vi "LabviewMonitoringApplicationFullDataFromCloud.vi"() -> ()   [LabVIEW 2024]
uses:
  <vilib>/Utility/error.llb/Trim Whitespace One-Sided.vi
  <vilib>/Instr/_visa.llb/VISA Configure Serial Port (Instr).vi
  <vilib>/Utility/file.llb/Read Delimited Spreadsheet (DBL).vi
  <vilib>/regexp/Match Regular Expression.xnode
  <vilib>/httpClient/LabVIEWHTTPClient.lvlib
  <vilib>/JDP Science/JSONtext/JSONtext.lvlib
panel:
  out "body":string
  out "CONTROL PANEL":enum32{"DASHBOARD", "Settings"}(tab)
  out "HISTORICAL DATA":dbl[][](graph)
  in  "To":string
  in  "From":string
  in  "Date":string
  in  "OK Button":bool
  in  "C/F":bool
  out "Pericol pentru sanatate":u32(colorbox)
  out "Disconfort sever":u32(colorbox)
  out "Disconfort moderat":u32(colorbox)
  out "Usor discomfort":u32(colorbox)
  out "Confortabil":u32(colorbox)
  out "Snapshot data":string
  out "Waveform Chart":T1(graph) caption="LIVE DATA"
  out "return count read":u32
  in  "STOP":bool=TRUE
  in  "milliseconds to wait":u32=1000
  out "VISA resource name out read":refnum<visa-resource-name>="COM32"
  in  "Start Measurement":bool=TRUE
  out "READ BUFFER":string
  out "Prog. Cnt":i64
  out "AdcValue":dbl
  out "R0 value (kOHm)":dbl(slide) scale=0.0..10.0 scale format="%.2f"
  out "Volatge":dbl(knob) scale=0.0..3.3
  out "Temperature °C":dbl(slide) scale=0.0..100.0 scale format="%#.2g"
  out "Humidity %":dbl(knob) scale=0.1..100.0 scale format="%#.2g"
  out "Heat Index":dbl(slide) scale=0.0..100.0
  out "iPPM_Smoke":i64(slide) scale=0.0..500.0
  out "iPPM_LPG":i64(slide) scale=0.0..100.0
  out "iPPM_CO":i64(slide) scale=0.0..400.0
  in  "Live Data / Historical Data":bool=TRUE
  in  "Temperature":bool=TRUE
  in  "Humidity":bool=TRUE
  in  "PMM_CO":bool=TRUE
  in  "HeatIndex":bool=TRUE
  in  "PMM_LPG":bool=TRUE
  in  "PMM_Smoke":bool=TRUE
  in  "Save file":bool
  in  "file path (use dialog)":path
  out "ITU":dbl format="%#.2g"
  in  "file path (dialog if empty)":path
  out "error out read  from VISA":errorcluster={"status"=TRUE, "code"=-1073807339, "source"="VISA Read in LabviewMonitoringApplication.vi"}
  in  "VISA resource name":refnum<visa-resource-name>="COM32"
  in  "Enable Termination\nChar (T)":bool=TRUE
  in  "timeout (ms)":u32=10000
  in  "baud rate (115200)":u32=115200
  in  "byte count":u32=100
  in  "parity (0:none)":enum16{"None", "Odd", "Even", "Mark", "Space"}(ring)
  in  "data bits (8)":u16=8 min=5 max=8 step=1
  in  "termination char\n(0xA = '\\n' = LF)":u8=10 format="%.0x"
  in  "flow control (0:none)":u16(ring) items=["None", "XON/XOFF", "RTS/CTS", "XON/XOFF & RTS/CTS", "DTR/DSR", "XON/XOFF & DTR/DSR"]
  in  "stop bits (10: 1 bit)":u16(ring)=10 items=["1.0"=10, "1.5"=15, "2.0"=20]
  out "error writing file":errorcluster
  out "Snapshot line":string
  out "Redirrect URL":string
  out "URL":string
  out "Data":string
  out "Header":string
  # "Select signals (for live data)"
  # "FILE HANDLING"
  # "VISA CONFIG"
  # "HTTP\nHANDLER"
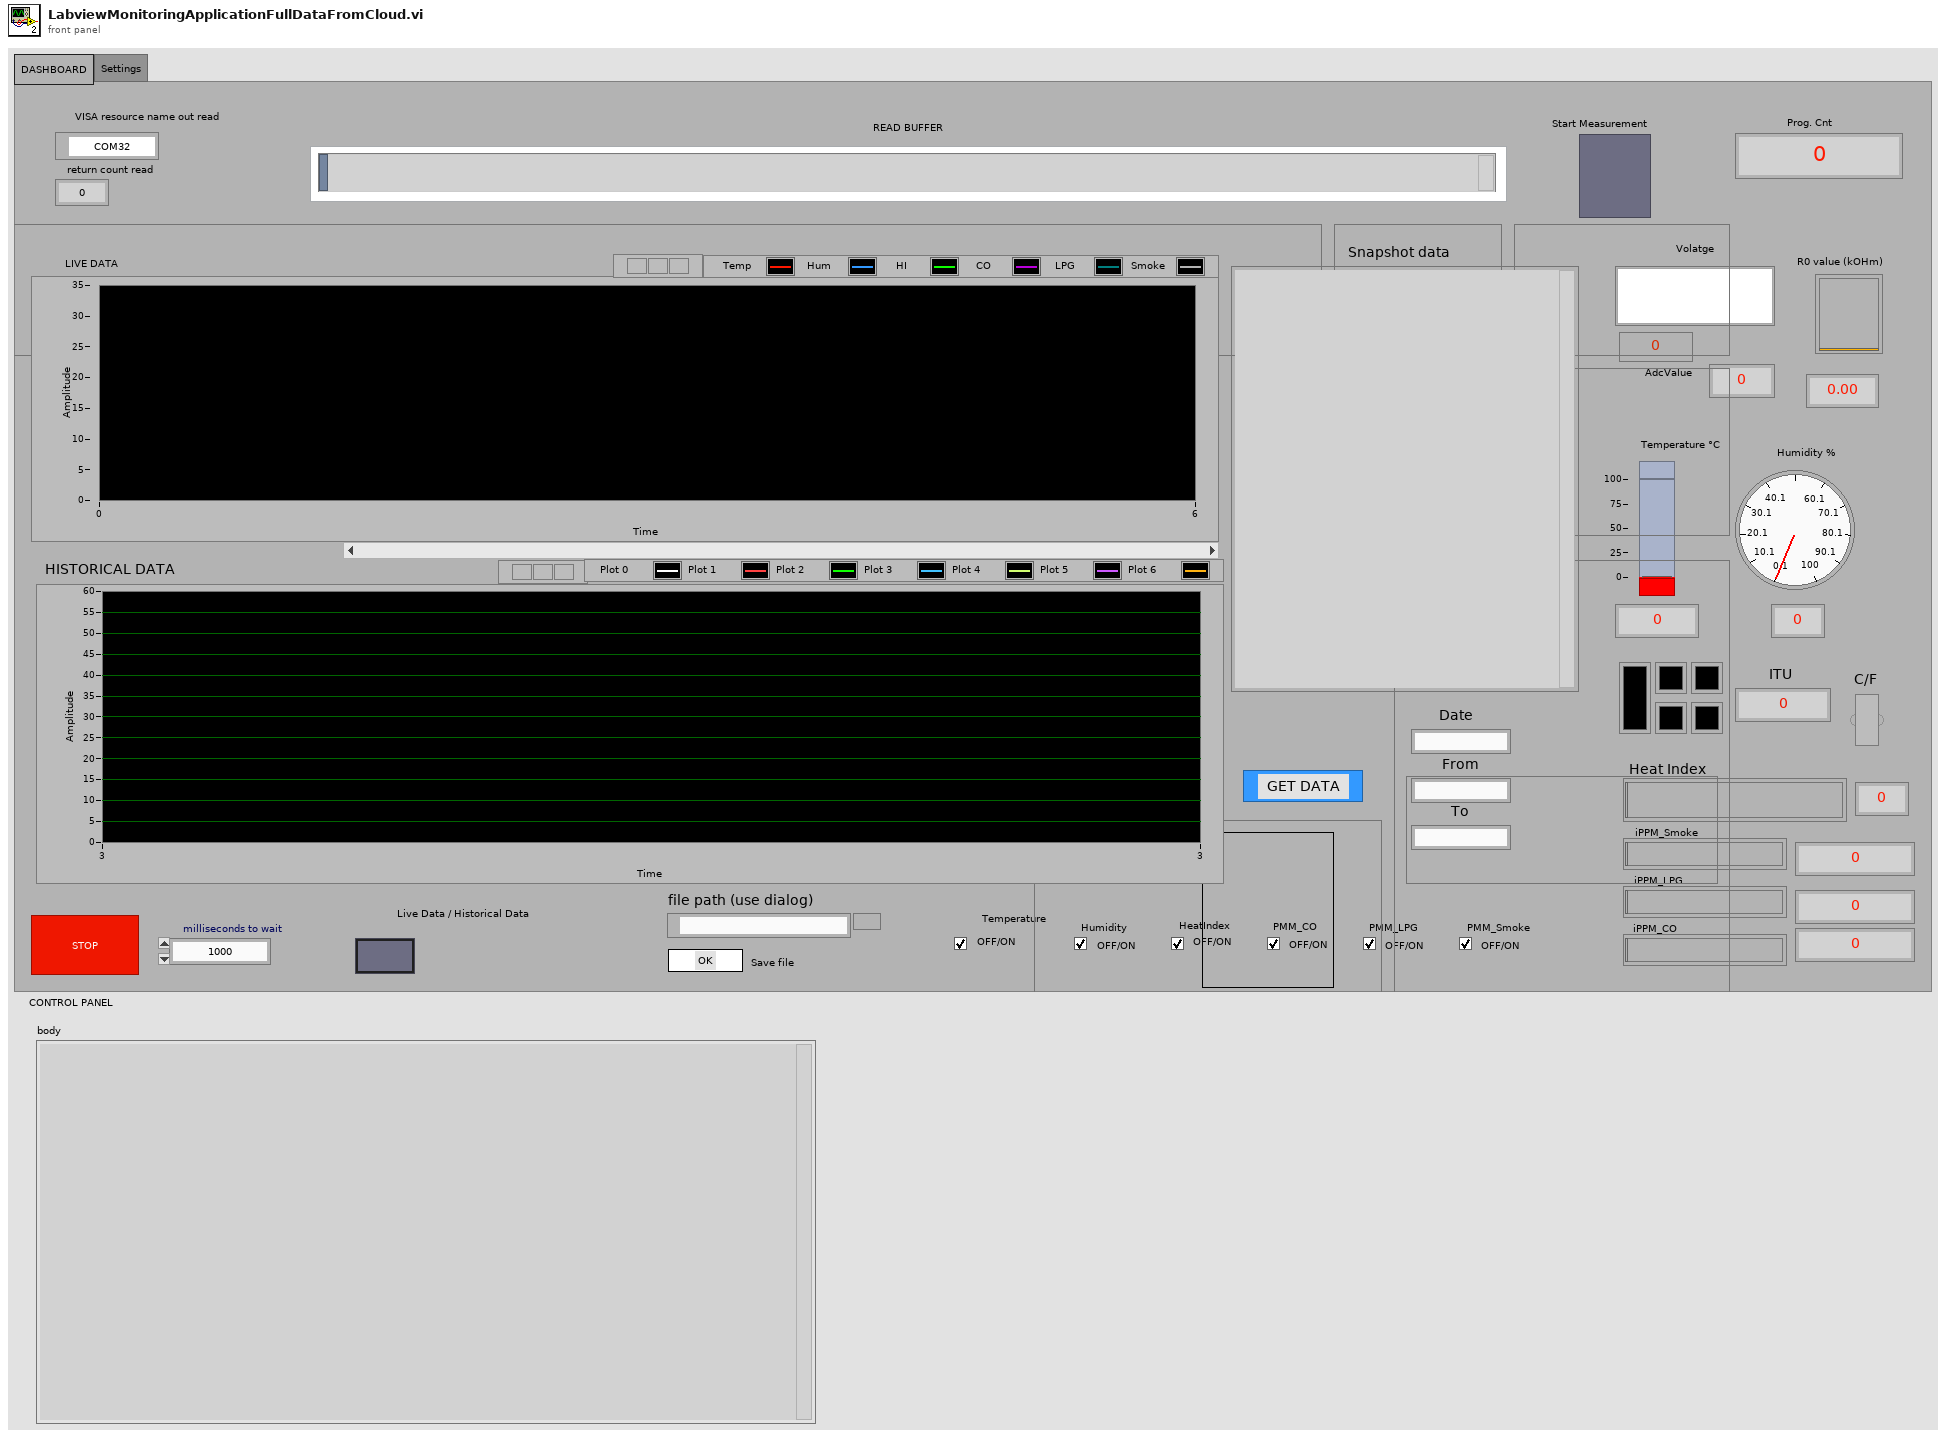
[diagram p1: front panel]
types:
  T1 = cluster{"Temperature °C ":dbl, "Humidity %":dbl, "Heat Index":dbl, "iPPM_CO":dbl, "iPPM_LPG":dbl, "iPPM_Smoke":dbl}
  T2 = cluster{"timestamp":string, "temperature ":dbl, "heatIndex":dbl, "humidity":dbl, "iPPM_LPG":dbl, "iPPM_CO":dbl, "iPPM_Smoke":dbl, "adcMq2Voltage":dbl, "Ro":dbl, "adcRawValue":dbl}[]
  T3 = enum16{"open", "replace", "create", "open or create", "replace or create", "replace or create with confirmation"}
  T4 = cluster{"timestamp":string, "iPPM_LPG":dbl, "temperature":dbl, "humidity":dbl, "iPPM_CO":dbl, "iPPM_Smoke":dbl}
  T5 = typedef "LabVIEWHTTPClient.lvlib/ClientHandle.ctl" = refnum<k1>
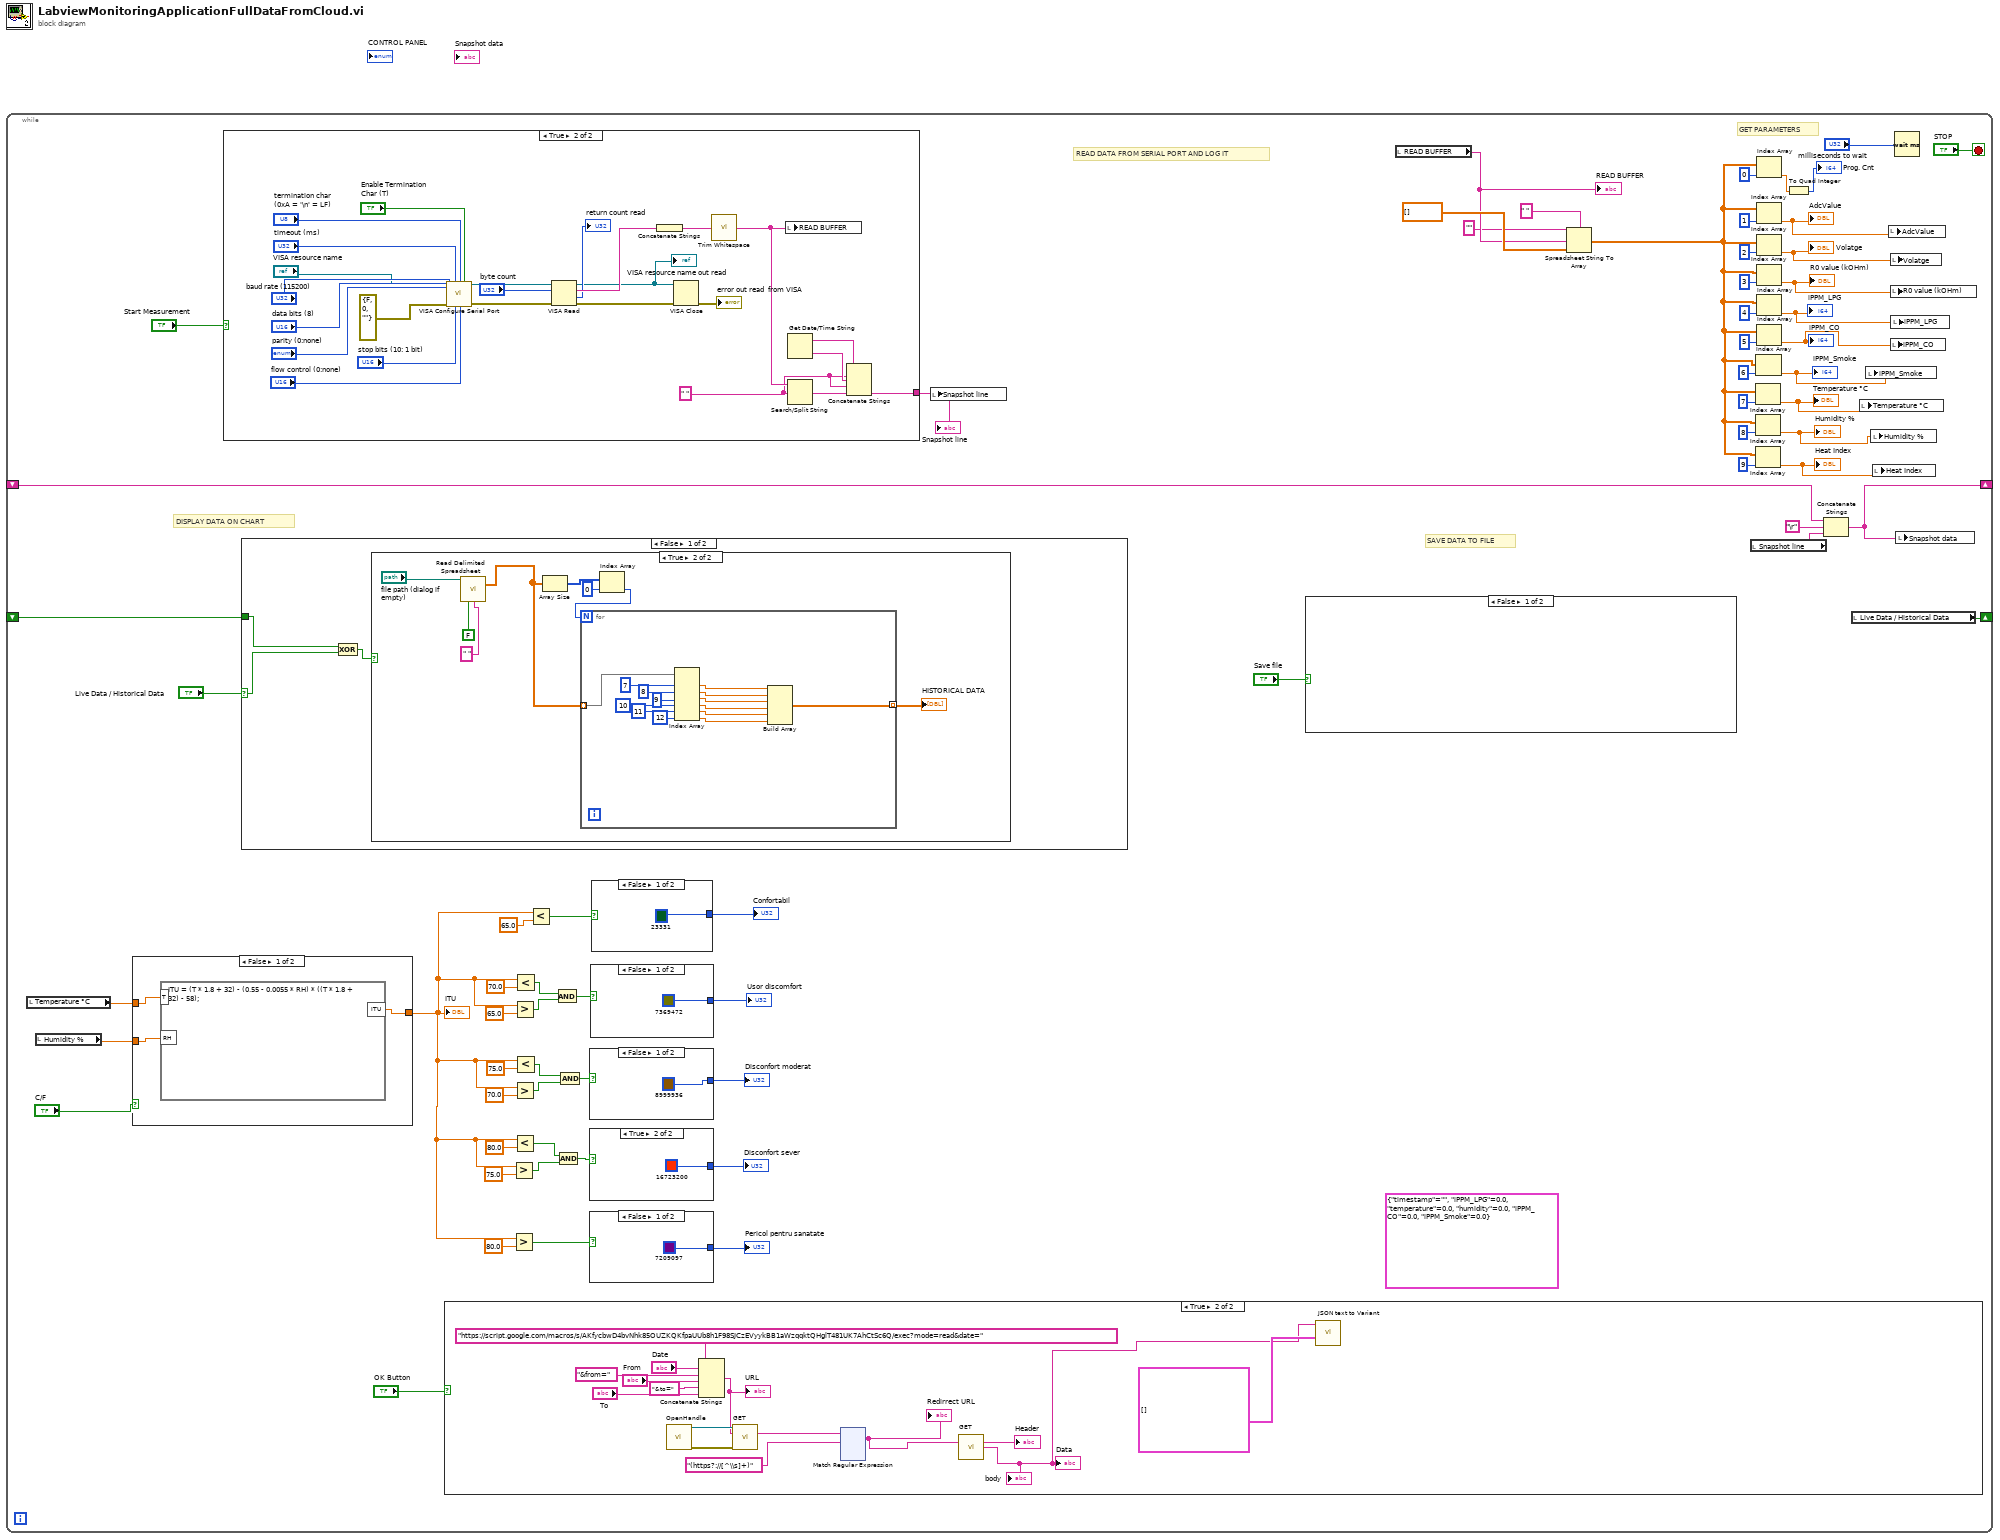
[diagram p0: block diagram]
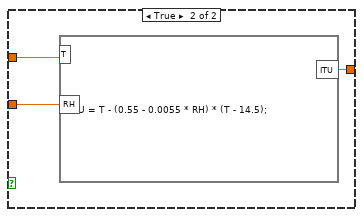
[diagram p3: hidden frame]
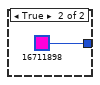
[diagram p4: hidden frame]
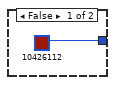
[diagram p5: hidden frame]
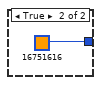
[diagram p6: hidden frame]
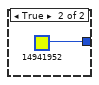
[diagram p7: hidden frame]
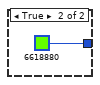
[diagram p8: hidden frame]
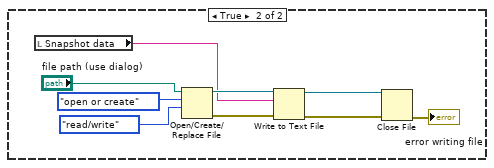
[diagram p9: hidden frame]
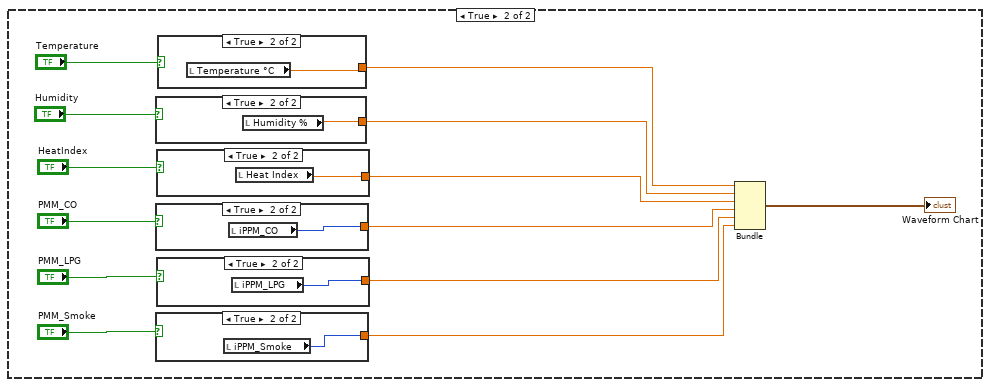
[diagram p11: hidden frame]
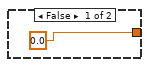
[diagram p12: hidden frame]
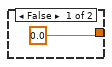
[diagram p13: hidden frame]
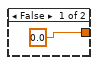
[diagram p14: hidden frame]
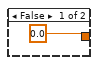
[diagram p15: hidden frame]
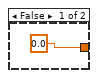
[diagram p16: hidden frame]
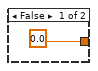
[diagram p17: hidden frame]
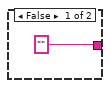
[diagram p18: hidden frame]
diagram:
  n1 = while {
    shift-right: [w34] -> _
    shift-left: _ -> [w35]
    shift-right: [w31] -> _
    shift-left: _ -> [w30]
    stop <- "STOP" stop-if-true
    (unwired) T4 {"timestamp"="", "iPPM_LPG"=0.0, "temperature"=0.0, "humidity"=0.0, "iPPM_CO"=0.0, "iPPM_Smoke"=0.0}
    # "SAVE DATA TO FILE"
    # "DISPLAY DATA ON CHART"
    # "READ DATA FROM SERIAL PORT AND LOG IT"
    # "GET PARAMETERS"
    n2 = local read "Temperature °C"() -> (w28:dbl)
    n3 = local read "Humidity %"() -> (w29:dbl)
    n4 = case shown="False" "C/F" {
      tunnel: w29 -> [w201 w205]
      tunnel: w28 -> [w202 w204]
      tunnel: [w200 w203] -> w3
      frame False {
        n5 = formula code="ITU = (T * 1.8 + 32) - (0.55 - 0.0055 * RH) * ((T * 1.8 + 32) - 58);"("T"=w202, "RH"=w201) -> ("ITU"=w200:dbl)
      }
      frame True {
        n6 = formula code="ITU = T - (0.55 - 0.0055 * RH) * (T - 14.5);"("T"=w204, "RH"=w205) -> ("ITU"=w203:dbl)
      }
    }
    "ITU" <- w3
    n7 = case shown="True" "Start Measurement" {
      tunnel: ["" w279] -> w33
      frame False {
      }
      frame True {
        w277 = " "
        n8 = call-poly "VISA Configure Serial Port"("VISA resource name"="VISA resource name", "timeout (10sec)"="timeout (ms)", "termination char\n(0xA = '\\n' = LF)"="termination char\n(0xA = '\\n' = LF)", "Enable Termination\nChar (T)"="Enable Termination\nChar (T)", "baud rate (9600)"="baud rate (115200)", "data bits (8)"="data bits (8)", "parity (0:none)"="parity (0:none)", "error in (no error)"=errorcluster {"status"=FALSE, "code"=0, "source"=""}, "stop bits (10: 1 bit)"="stop bits (10: 1 bit)", "flow control (0:none)"="flow control (0:none)") -> ("VISA resource name out"=w293:refnum<visa-resource-name>, "error out"=w292:errorcluster)  [unwired: 4 in]
        n9 = VISA Read(VISA resource name=w293, byte count="byte count", error in (no error)=w292) -> (VISA resource name out=w282:refnum<visa-resource-name>, read buffer=w291:string, return count=→"return count read":u32, error out=w283:errorcluster)
        "VISA resource name out read" <- w282
        n10 = Concatenate Strings(w291) -> (w288:string)
        n11 = VISA Close(VISA resource name=w282, error in (no error)=w283) -> (error out=→"error out read  from VISA":errorcluster)
        n12 = call <vilib>:"Trim Whitespace.vi"("string"=w288) -> ("trimmed string"=w280:string)  [unwired: 1 in]
        n13 = local write "READ BUFFER"(w280) -> ()
        n14 = Search/Split String(string=w280, search string/char (-)=w277) -> (match + rest of string=w281:string)  [unwired: 1 in, 2 out]
        n15 = Get Date/Time String() -> (date string=w276:string, time string=w278:string)  [unwired: 3 in]
        n16 = Concatenate Strings(w276, w277, w278, w277, w281) -> (w279:string)
      }
    }
    "Snapshot line" <- w33
    n17 = case shown="False" "Live Data / Historical Data" {
      selector: "Live Data / Historical Data" -> [w226 _]
      tunnel: w30 -> [w227 _]
      frame False {
        n18 = Exclusive Or(1:w226, 2:w227) -> (0:w225:bool)
        n19 = case shown="True" w225 {
          frame False {
          }
          frame True {
            n20 = call-poly <vilib>:"Read Delimited Spreadsheet.vi"("file path (dialog if empty)"="file path (dialog if empty)", "transpose? (F)"=FALSE, "delimiter (\\t)"=" ") -> ("all rows"=w229:dbl[][])  [unwired: 7 in, 5 out]
            n21 = Array Size(array=w229) -> (size(s)=w231:i32[])
            n22 = Index Array(array=w231, index=0) -> (element=w230:i32)
            n23 = for {
              N: w230 -> [_]
              tunnel: w229 -> [w243] mode=indexing
              tunnel: [w236] -> w228 mode=indexing
              n24 = Index Array(array=w243, index #1=7 ("index"), index #2=8 ("index"), index #3=9 ("index"), index #4=10 ("index"), index #5=11 ("index"), index #6=12 ("index")) -> (element #1=w242:dbl, element #2=w241:dbl, element #3=w240:dbl, element #4=w239:dbl, element #5=w238:dbl, element #6=w237:dbl)
              n25 = Build Array(w242, w241, w240, w239, w238, w237) -> (w236:dbl[])
            }
            "HISTORICAL DATA" <- w228
          }
        }
      }
      frame True {
        n26 = case shown="True" "Humidity" {
          tunnel: [0.0 w272] -> w255
          frame False {
          }
          frame True {
            n27 = local read "Humidity %"() -> (w272:dbl)
          }
        }
        n28 = case shown="True" "PMM_CO" {
          tunnel: [0.0 w268] -> w253
          frame False {
          }
          frame True {
            n29 = local read "iPPM_CO"() -> (w268:i64)
          }
        }
        n30 = case shown="True" "PMM_Smoke" {
          tunnel: [0.0 w264] -> w251
          frame False {
          }
          frame True {
            n31 = local read "iPPM_Smoke"() -> (w264:i64)
          }
        }
        n32 = case shown="True" "HeatIndex" {
          tunnel: [0.0 w270] -> w254
          frame False {
          }
          frame True {
            n33 = local read "Heat Index"() -> (w270:dbl)
          }
        }
        n34 = case shown="True" "PMM_LPG" {
          tunnel: [0.0 w266] -> w252
          frame False {
          }
          frame True {
            n35 = local read "iPPM_LPG"() -> (w266:i64)
          }
        }
        n36 = case shown="True" "Temperature" {
          tunnel: [0.0 w274] -> w261
          frame False {
          }
          frame True {
            n37 = local read "Temperature °C"() -> (w274:dbl)
          }
        }
        n38 = Bundle("Temperature °C"=w261, "Humidity %"=w255, "Heat Index"=w254, "iPPM_CO"=w253, "iPPM_LPG"=w252, "iPPM_Smoke"=w251) -> (→"Waveform Chart":T1)  [unwired: 1 in]
      }
    }
    n39 = case shown="True" "OK Button" {
      frame False {
      }
      frame True {
        n40 = call <vilib>:"OpenHandle.vi"() -> ("client handle out"=w82:T5, "error out"=w81:errorcluster)  [unwired: 14 in]
        n41 = Concatenate Strings("https://script.google.com/macros/s/AKfycbwD4bvNhk85OUZKQKfpaUUb8h1F98SJCzEVyykBB1aWzqqktQHglT481UK7AhCtSc6Q/exec?mode=read&date=" ("url"), "Date", "&from=" ("string"), "From", "&to=" ("string"), "To") -> (w80:string)
        "URL" <- w80
        n42 = call <vilib>:"GET.vi"("client handle"=w82, "url"=w80, "error in (no error)"=w81) -> ("headers"=w72:string)  [unwired: 9 in, 3 out]
        n43 = xnode "Match Regular Expression"("input string"=w72, "regular expression"="(https?://[^\\s]+)") -> ("whole match"=w73:string)  [unwired: 4 in, 4 out]
        "Redirrect URL" <- w73
        n44 = call <vilib>:"GET.vi"("url"=w73) -> ("headers"=→"Header":string, "body"=w68:string)  [unwired: 11 in, 2 out]
        "Data" <- w68
        "body" <- w68
        n45 = call <vilib>:"JSON text to Variant.vi"("Data Type"=T2 [], "JSON"=w68) -> ()  [unwired: 8 in, 2 out]
      }
    }
    n46 = Greater?(x=w3, y=75.0) -> (0:w15:bool)
    n47 = Greater?(x=w3, y=80.0) -> (0:w20:bool)
    n48 = Greater?(x=w3, y=65.0) -> (0:w12:bool)
    n49 = Greater?(x=w3, y=70.0) -> (0:w14:bool)
    n50 = Less?(x=w3, y=80.0) -> (x < y?=w16:bool)
    n51 = Less?(x=w3, y=70.0) -> (x < y?=w11:bool)
    n52 = Less?(x=w3, y=75.0) -> (x < y?=w13:bool)
    n53 = Less?(x=w3, y=65.0 ("x")) -> (x < y?=w27:bool)
    n54 = And(x=w11, y=w12) -> (x .and. y?=w19:bool)
    n55 = And(x=w16, y=w15) -> (x .and. y?=w17:bool)
    n56 = And(x=w13, y=w14) -> (x .and. y?=w18:bool)
    n57 = case shown="False" w18 {
      tunnel: [u32 8999936 ("Pericol pentru sanatate 2") u32 16751616 ("Pericol pentru sanatate 2")] -> w23
      frame False {
      }
      frame True {
      }
    }
    "Disconfort moderat" <- w23
    n58 = case shown="True" w17 {
      tunnel: [u32 10426112 ("Pericol pentru sanatate 2") u32 16723200 ("Pericol pentru sanatate 2")] -> w24
      frame False {
      }
      frame True {
      }
    }
    "Disconfort sever" <- w24
    n59 = case shown="False" w20 {
      tunnel: [u32 7209097 ("Pericol pentru sanatate 2") u32 16711898 ("Pericol pentru sanatate 2")] -> w25
      frame False {
      }
      frame True {
      }
    }
    "Pericol pentru sanatate" <- w25
    n60 = case shown="False" w19 {
      tunnel: [u32 7369472 ("Pericol pentru sanatate 2") u32 14941952 ("Pericol pentru sanatate 2")] -> w22
      frame False {
      }
      frame True {
      }
    }
    "Usor discomfort" <- w22
    n61 = case shown="False" w27 {
      tunnel: [u32 23331 ("Pericol pentru sanatate 2") u32 6618880 ("Pericol pentru sanatate 2")] -> w26
      frame False {
      }
      frame True {
      }
    }
    "Confortabil" <- w26
    n62 = local write "Snapshot line"(w33) -> ()
    n63 = case shown="False" "Save file" {
      frame False {
      }
      frame True {
        n64 = local read "Snapshot data"() -> (w218:string)
        n65 = Open/Create/Replace File(file path (use dialog)="file path (use dialog)", operation (0:open)=T3."open or create", access (0:read/write)=enum16{"read/write", "read-only", "write-only"}."read/write") -> (refnum out=w223:refnum<file>, error out=w222:errorcluster)  [unwired: 3 in, 1 out]
        n66 = Write to Text File(file (use dialog)=w223, text=w218, error in=w222) -> (refnum out=w220:refnum<file>, error out=w221:errorcluster)  [unwired: 1 in, 1 out]
        n67 = Close File(refnum=w220, error in=w221) -> (error out=→"error writing file":errorcluster)  [unwired: 1 out]
      }
    }
    n68 = local read "READ BUFFER"() -> (w63:string)
    "READ BUFFER" <- w63
    n69 = Spreadsheet String To Array(delimiter (Tab)=" ", format string="", spreadsheet string=w63, array type (2D Dbl)=dbl[] []) -> (array=w49:dbl[])
    n70 = local read "Snapshot line"() -> (w32:string)
    n71 = Index Array(array=w49, index=7) -> (element=w41:dbl)
    "Temperature °C" <- w41
    n72 = Index Array(array=w49, index=8) -> (element=w42:dbl)
    "Humidity %" <- w42
    n73 = Index Array(array=w49, index=9) -> (element=w43:dbl)
    "Heat Index" <- w43
    n74 = Index Array(array=w49, index=6) -> (element=w40:dbl)
    "iPPM_Smoke" <- w40
    n75 = Index Array(array=w49, index=0) -> (element=w60:dbl)
    n76 = Index Array(array=w49, index=1) -> (element=w48:dbl)
    "AdcValue" <- w48
    n77 = Index Array(array=w49, index=2) -> (element=w47:dbl)
    "Volatge" <- w47
    n78 = Index Array(array=w49, index=3) -> (element=w46:dbl)
    "R0 value (kOHm)" <- w46
    n79 = Index Array(array=w49, index=4) -> (element=w45:dbl)
    "iPPM_LPG" <- w45
    n80 = Index Array(array=w49, index=5) -> (element=w44:dbl)
    "iPPM_CO" <- w44
    n81 = To Quad Integer(1:w60) -> (0:→"Prog. Cnt":i64)
    n82 = Concatenate Strings(w35, "\r", w32) -> (w34:string)
    n83 = local read "Live Data / Historical Data"() -> (w31:bool)
    n84 = local write "Temperature °C"(w41) -> ()
    n85 = local write "iPPM_Smoke"(w40) -> ()
    n86 = local write "Humidity %"(w42) -> ()
    n87 = local write "Heat Index"(w43) -> ()
    n88 = local write "AdcValue"(w48) -> ()
    n89 = local write "Volatge"(w47) -> ()
    n90 = local write "R0 value (kOHm)"(w46) -> ()
    n91 = local write "iPPM_CO"(w44) -> ()
    n92 = local write "iPPM_LPG"(w45) -> ()
    n93 = Wait (ms)(milliseconds to wait="milliseconds to wait") -> ()  [unwired: 1 out]
    n94 = local write "Snapshot data"(w34) -> ()
  }
